vi "Read Aborted.vi"(8 "error in (no error)":errorcluster, 11 "AFM_Driver in":refnum<class "AFM_Driver.lvclass">) -> (0 "error out":errorcluster, 2 "Aborted?":bool, 3 "AFM_Driver out":refnum<class "AFM_Driver.lvclass">)   [LabVIEW 2019, in "AFM_Driver.lvclass"]
uses:
  AFM_Driver.lvclass
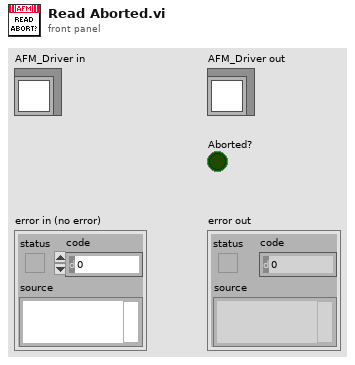
[diagram p1: front panel]
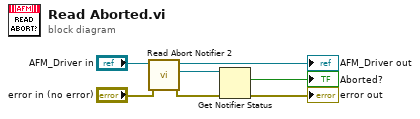
[diagram p0: block diagram]
diagram:
  n1 = call-dynamic "Read Abort Notifier 2.vi"("error in (no error)"="error in (no error)", "AFM_Driver in"="AFM_Driver in") -> ("error out"=w1:errorcluster, "Abort Notifier"=w4:refnum<notifier>, "AFM_Driver out"=→"AFM_Driver out":refnum<class "AFM_Driver.lvclass">)  [unwired: 7 in]
  n2 = Get Notifier Status(notifier=w4, error in (no error)=w1) -> (current notification=→"Aborted?":bool, error out=→"error out":errorcluster)  [unwired: 3 out]
